vi "Dashboard Main.vi"() -> ()   [LabVIEW 2013]
uses:
  <vilib>/event_ctls.llb/eventvkey.ctl
  <vilib>/Rock Robotics/WPI/Dashboard/WPI_DashboardLogging Global.vi
  <vilib>/Utility/config.llb/Write Key (String).vi
  <vilib>/Utility/config.llb/Write Key (I32).vi
  <vilib>/Utility/config.llb/NI_LVConfig.lvlib
panel:
  out "Image Message":string="Timeout in Camera Communications"
  in  "Rec Mode":enum32{"Stop", "Record", "Playback"}(radio)
  in  "Dashboard Tab":T1(tab)
  out "Error":bool
  in  "Camera Settings":T2={"Frame Rate"=30, "Compression"=30, "Size"=1} {"Frame Rate" scale=1.0..30.0; "Size" items=["640x480", "320x240", "160x120"]}
  out "MotorSliders R":cluster{"MotorSlide1":dbl, "MotorSlide2":dbl} {"MotorSlide2" scale=-1.0..1.0 scale format="%#_2e"; "MotorSlide1" scale=-1.0..1.0 scale format="%#_2e"}
  out "MotorChart R":cluster{"Numeric":dbl, "Numeric":dbl}(graph)
  out "MotorSliders L":T3 {"MotorSlide4 2" scale=0.0..14.0 scale format="%#_2e"; "MotorSlide2" scale=-1.0..1.0 scale format="%#_2e"; "MotorSlide1" scale=-1.0..1.0 scale format="%#_2e"}
  out "MotorChart L":T4(graph)
  out "JS1 Z":dbl(slide) scale=-1.0..1.0 scale format="%#_2e"
  out "Joystick 1":cluster{"X":dbl, "Y":dbl}[](graph)
  out "JS Buttons 1":T5
  out "JS2 Z":dbl(slide) scale=-1.0..1.0 scale format="%#_2e"
  out "Joystick 2":cluster{"X":dbl, "Y":dbl}[](graph)
  out "JS Buttons 2":T5
  out "Mode":T6(ring)=enum."Auto Disabled"
  out "Camera IP":string
  in  "DB Camera Config":bool
  out "fps":dbl format="%#.1g"
  out "Mbps":dbl format="%#.1g"
  out "Mbps 2":bool
  in  "Test Slider":dbl(slide) scale=0.0..100.0 scale format="%#_3g"
  in  "On/Off":bool caption="Solenoid"
  in  "Test Name":u16(ring) items=["Select the test to run...", "Example Test", "-------------------------------", "List of tests is built in robot code.", "Replace with your own automated tests."]
  in  "Test Tree":string(tree)
  in  "Motor":cluster{"Value":dbl, "Enable":bool} {"Value" scale=-1.0..1.0 scale format="%#_3g"}
  out "Progress":T7 {"Test Progress" scale=0.0..100.0}
  in  "Rev/Fwd":cluster{"Forward":bool, "Reverse":bool}
  in  "Test Ring":u16(ring) items=["Auto", "Fixed indoor", "Fixed outdoor 1", "Fixed outdoor 2", "Fixed fluorescent 1", "Fixed fluorescent 2", "Hold current"]
  in  "Listbox":i32(listbox)
  out "Tree":string(tree)
  out "Errors":T8(array[cluster])
  out "Camera Image":T9(plugin-control)
  in  "Enable":bool
  # "Left"
  # "Front"
  # "Right"
  # "Battery"
  # "Customize by placing controls and indicators here and name to\nmatch Dashboard Variables on robot."
  # "This tab is a great place for autonomous settings and validation.\nCustomize by placing controls and indicators here and name to\nmatch Dashboard Variables on robot."
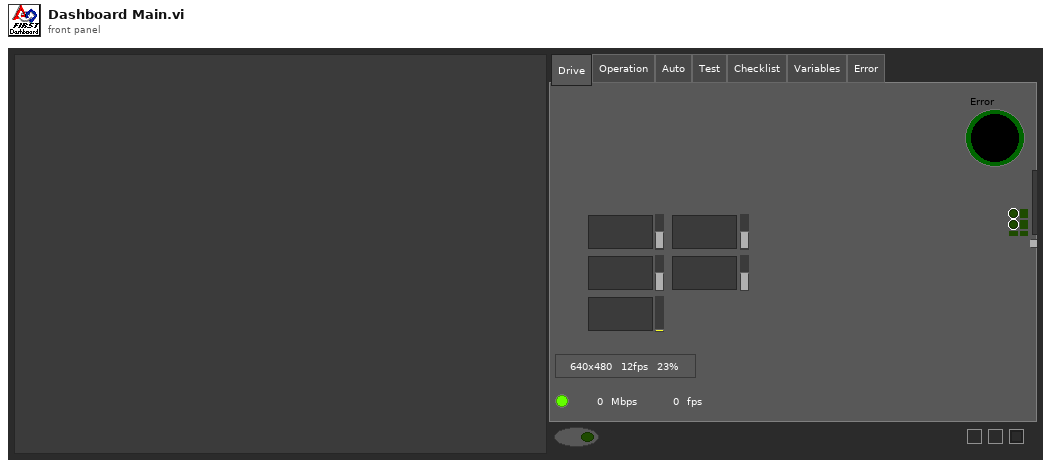
[diagram p1: front panel]
types:
  T1 = enum32{"Drive", "Operation", "Auto", "Test", "Checklist", "Variables", "Error"}
  T2 = cluster{"Frame Rate":i32, "Compression":i32, "Size":u16}
  T3 = cluster{"MotorSlide1":dbl, "MotorSlide2":dbl, "MotorSlide4 2":dbl}
  T4 = cluster{"Numeric":dbl, "Numeric":dbl, "Battery":sgl}
  T5 = cluster{bool, bool, bool, bool, bool, bool, bool, bool, bool, bool, bool, bool}
  T6 = enum8{"Tele-Op Disabled", "Tele-Op Enabled", "Auto Disabled", "Auto Enabled", "Test Disabled", "Test Enabled", ""}
  T7 = cluster{"Test Progress":u8, "Test Progress Text":string}
  T8 = cluster{"status":bool, "code":i32, "location":string, "source":string}[]
  T9 = typedef "IMAQ Image.ctl" = refnum<image>
  T10 = enum32{"Drive", "Operation", "Auto", "Test", "Checklist", "Variables"}
  T11 = typedef "Image Type" = u32
  T12 = cluster{"Digital Inputs":bool[], "Digital Outputs":bool[]}
  T13 = cluster{"Competition mode":bool, "Robot Link":bool, "Autonomous":bool, "Enabled":bool, "E-Stop":bool, "Simulated":bool, "TestMode":bool, "Docked Window":bool}
  T14 = cluster{"Boolean":bool, "Numeric":i32, "String":string, "String":string}[]
  T15 = cluster{"Boolean Array[0]":bool, "Boolean Array[1]":bool, "Boolean Array[2]":bool, "Boolean Array[3]":bool, "Boolean Array[4]":bool, "Boolean Array[5]":bool, "Boolean Array[6]":bool, "Boolean Array[7]":bool, "Boolean Array[8]":bool, "Boolean Array[9]":bool, "Boolean Array[10]":bool, "Boolean Array[11]":bool}
  T16 = typedef "NI_LVConfig.lvlib/Config Data RefNum.ctl" = refnum<k1>
  T17 = typedef "eventvkey.ctl" = enum16{"ASCII", "Enter", "Return", "Shift", "Ctrl", "Alt", "Cmd", "Opt", "Caps", "NumLock", "Clear", "Break", "Up", "Down", "Left", "Right", "Insert", "Delete", "Home", "End", "PageUp", "PageDown", "Escape", "Help", "Pause", "ScrollLock", "F1", "F2", "F3", "F4", "F5", "F6", "F7", "F8", "F9", "F10", "F11", "F12", "F13", "F14", "F15", "F16", "F17", "F18", "F19", "F20", "F21", "F22", "F23", "F24", "Play", "VolumeUp", "VolumeDown", "Mute", "Two Byte Char"}
  T18 = cluster{"Image Size":bool, "Image Type":bool, "Pixel Value":bool, "ROI Information":bool, "Zoom Factor":bool}
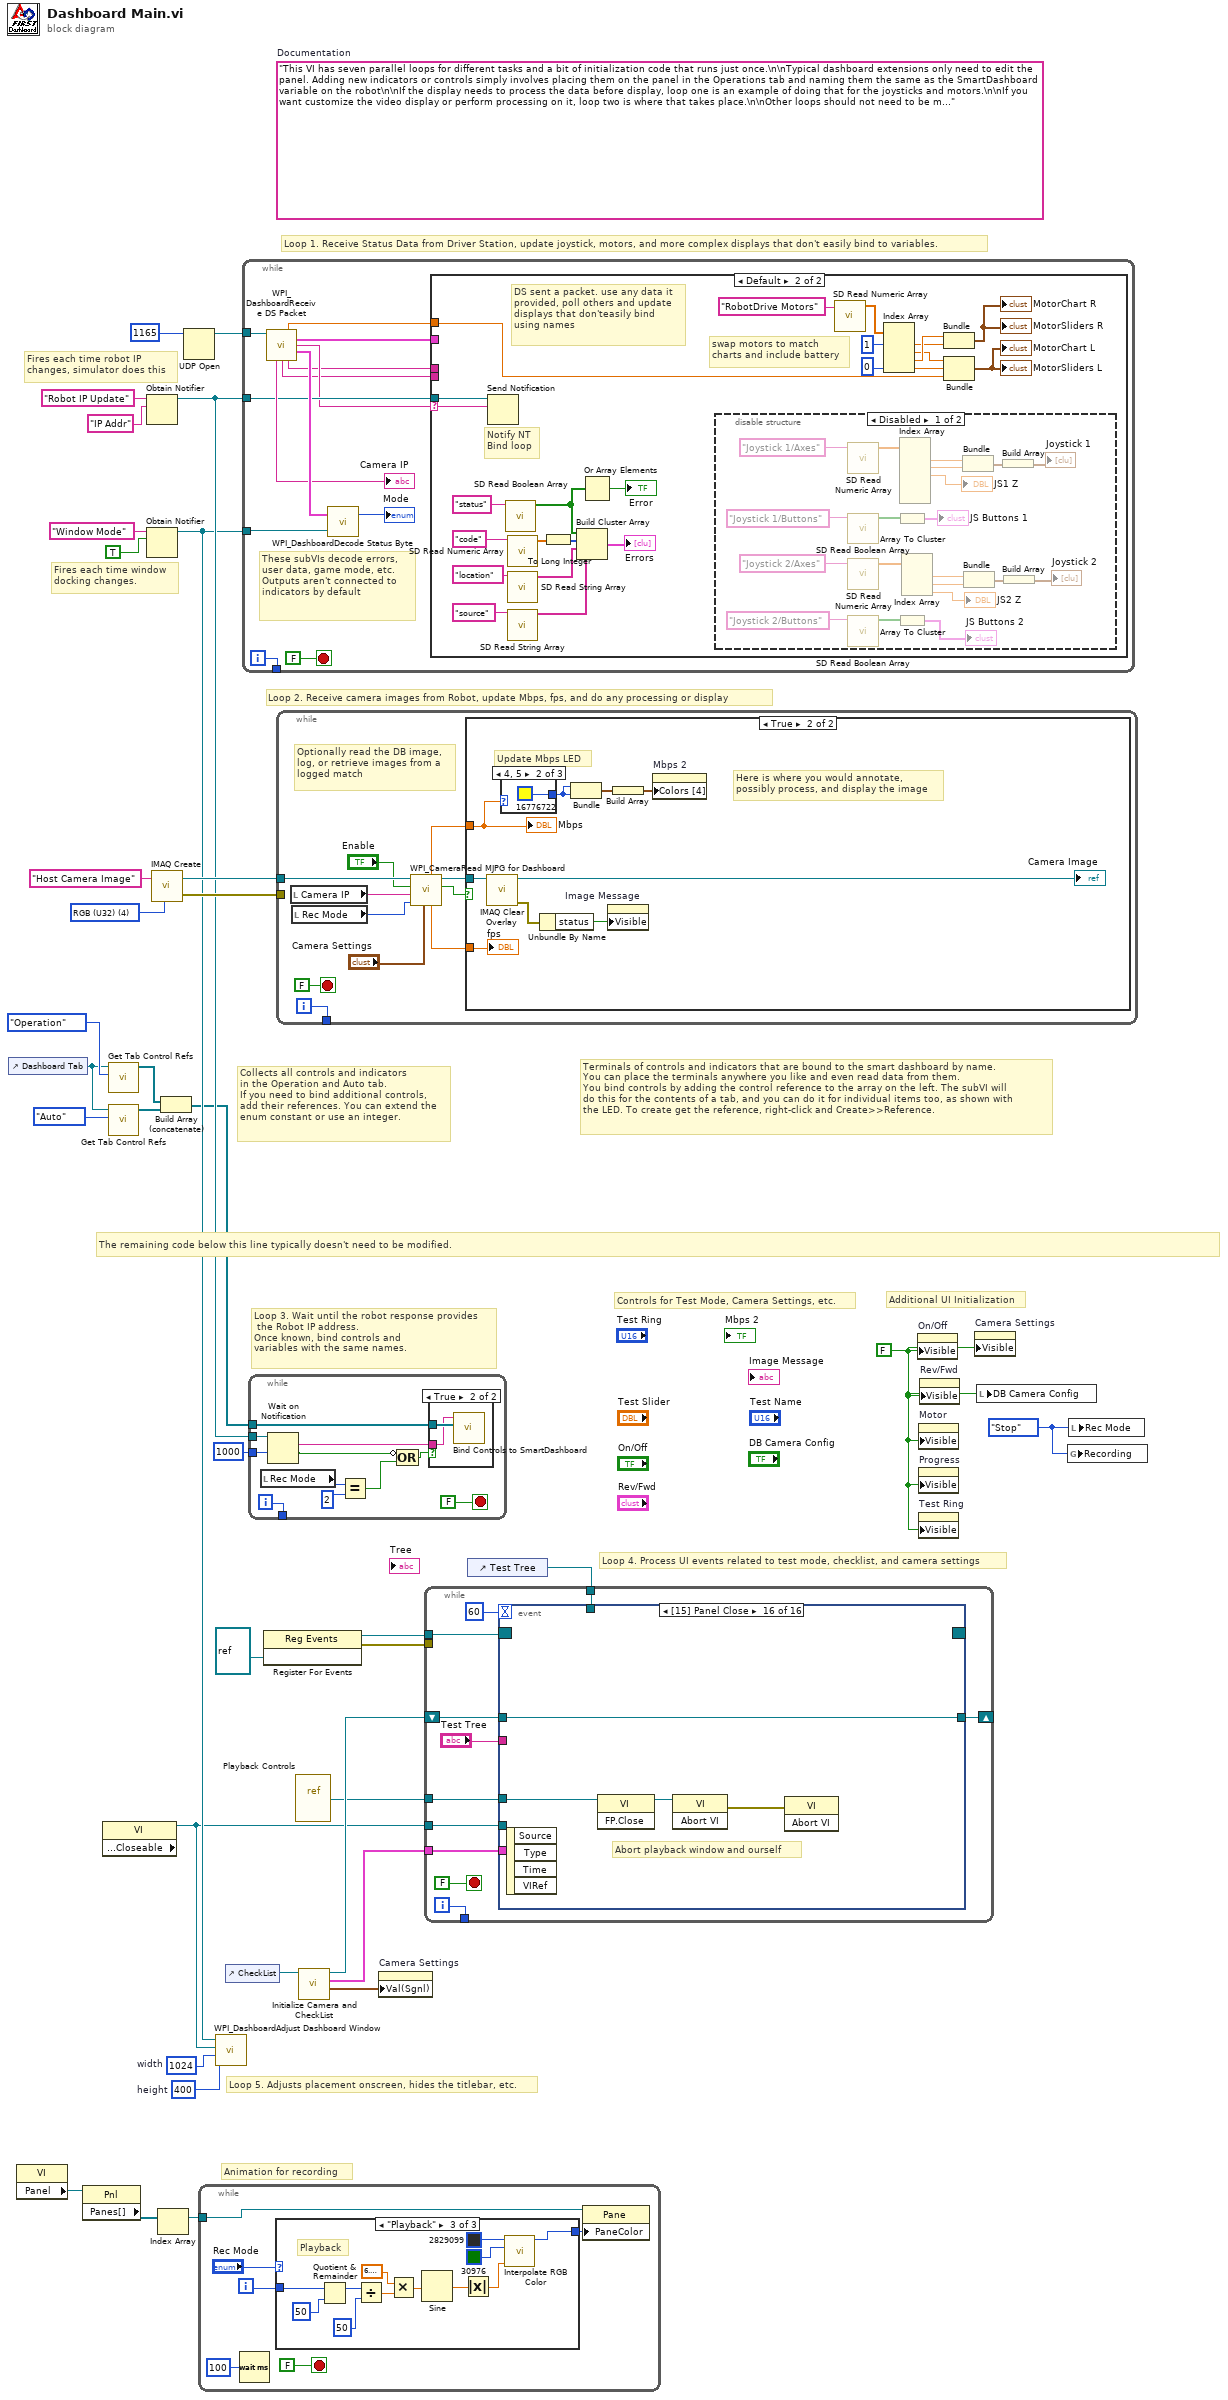
[diagram p0: block diagram]
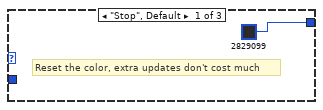
[diagram p2: hidden frame]
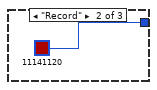
[diagram p3: hidden frame]
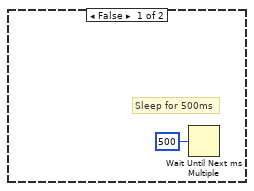
[diagram p5: hidden frame]
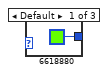
[diagram p6: hidden frame]
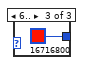
[diagram p7: hidden frame]
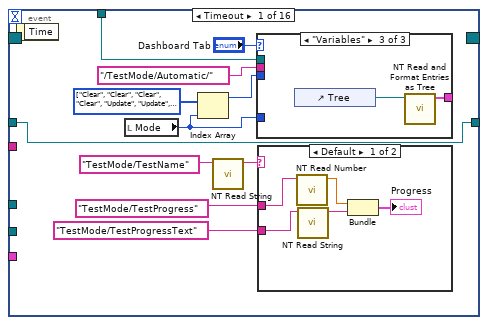
[diagram p8: hidden frame]
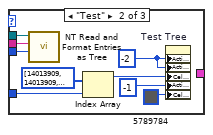
[diagram p10: hidden frame]
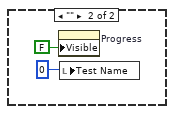
[diagram p11: hidden frame]
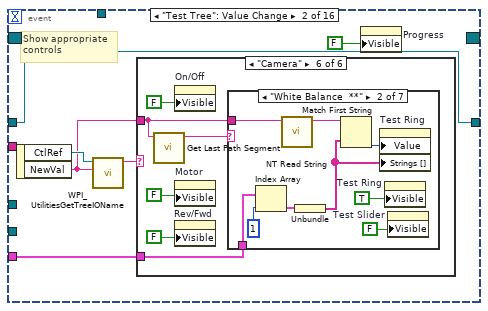
[diagram p12: hidden frame]
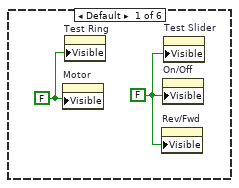
[diagram p13: hidden frame]
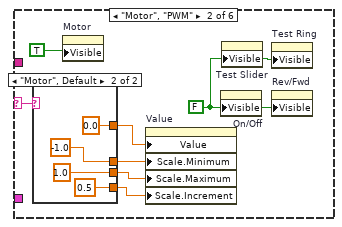
[diagram p14: hidden frame]
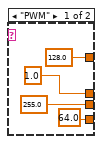
[diagram p15: hidden frame]
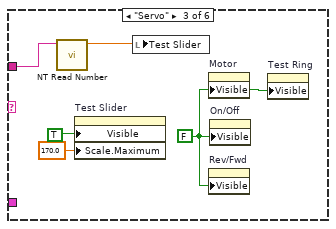
[diagram p16: hidden frame]
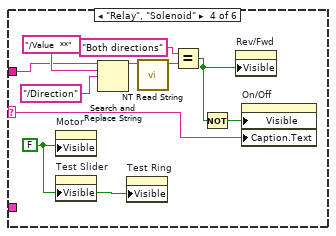
[diagram p17: hidden frame]
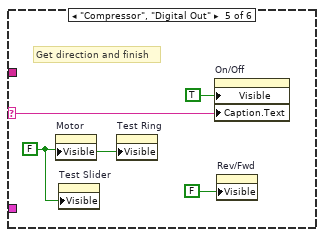
[diagram p18: hidden frame]
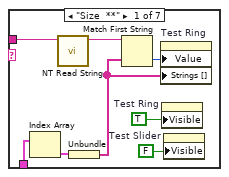
[diagram p19: hidden frame]
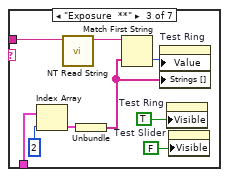
[diagram p20: hidden frame]
diagram:
  w7 = enum32{"Stop", "Record", "Playback"}."Stop" ("Rec Mode")
  w10 = 400  # height
  w11 = 1024  # width
  w24 = FALSE ("Visible")
  (unwired) "This VI has seven parallel loops for different tasks and a bit of initialization code that runs just once.\n\nTypical dashboard extensions only need to edit the panel. Adding new indicators or controls simply involves placing them on the panel in the Operations tab and naming them the same as the SmartDashboard variable on the robot\n\nIf the display needs to process the data before display, loop one is an example of doing that for the joysticks and motors.\n\nIf you want customize the video display or perform processing on it, loop two is where that takes place.\n\nOther loops should not need to be modified. They are pretty standard, and document the task they perform."  # Documentation
  w34 = T11 4 items=["Grayscale (U8)", "Grayscale (I16)", "Grayscale (SGL)", "Complex (CSG)", "RGB (U32)", "HSL (U32)", "RGB (U64)"] ("Image Type")
  # "Controls for Test Mode, Camera Settings, etc."
  # "Additional UI Initialization"
  # "Animation for recording"
  # "Fires each time robot IP\nchanges, simulator does this"
  # "Fires each time window\ndocking changes."
  # "Collects all controls and indicators\nin the Operation and Auto tab.\nIf you need to bind additional controls,\nadd their references. You can extend the\nenum constant or use an integer."
  # "The remaining code below this line typically doesn't need to be modified."
  # "Loop 4. Process UI events related to test mode, checklist, and camera settings"
  # "Terminals of controls and indicators that are bound to the smart dashboard by name.\nYou can place the terminals anywhere you like and even read data from them.\nYou bind controls by adding the control reference to the array on the left. The subVI will\ndo this for the contents of a tab, and you can do it for individual items too, as shown with\nthe LED. To create get the reference, right-click and Create>>Reference."
  # "Loop 3. Wait until the robot response provides\n the Robot IP address.\nOnce known, bind controls and\nvariables with the same names."
  # "Loop 5. Adjusts placement onscreen, hides the titlebar, etc."
  # "Loop 1. Receive Status Data from Driver Station, update joystick, motors, and more complex displays that don't easily bind to variables."
  # "Loop 2. Receive camera images from Robot, update Mbps, fps, and do any processing or display"
  n1 = control-ref of="Dashboard Tab"() -> (w5:refnum<vi>)
  n2 = property class="VI"() -> ("Panel"=w18:refnum<vi>)  [unwired: 2 in, 2 out]
  n3 = property class="Pnl"(reference=w18) -> ("Panes[]"=w19:refnum<vi>[])  [unwired: 1 in, 2 out]
  n4 = property class="VI" props=["Front Panel.Closeable"]() -> (reference out=w6:refnum<vi>)  [unwired: 2 in, 2 out]
  n5 = call <vilib>:"Get Tab Control Refs.vi"("Page Index"=T10."Operation" ("Dashboard Tab"), "TabControl in"=w5) -> ("ControlsOnPage"=w3:refnum<vi>[])  [unwired: 9 in]
  n6 = call <vilib>:"Get Tab Control Refs.vi"("Page Index"=T10."Auto" ("Dashboard Tab"), "TabControl in"=w5) -> ("ControlsOnPage"=w4:refnum<vi>[])  [unwired: 9 in]
  n7 = Obtain Notifier(name (unnamed)="Robot IP Update", notification data type="IP Addr" ("name (unnamed)")) -> (notifier out=w28:refnum<notifier>)  [unwired: 2 in, 2 out]
  n8 = Obtain Notifier(name (unnamed)="Window Mode", notification data type=TRUE) -> (notifier out=w9:refnum<notifier>)  [unwired: 2 in, 2 out]
  n9 = call "IMAQ Create"("Image Name"="Host Camera Image", "Image Type"=w34) -> ("New Image"=w32:T9, "error out"=w31:errorcluster)  [unwired: 2 in, 1 out]
  n10 = Index Array(array=w19) -> (element=w17:refnum<vi>)  [unwired: 1 in]
  n11 = Build Array (concatenate)(w3, w4) -> (w2:refnum<vi>[])
  n12 = UDP Open(11:u16 1165 ("port")) -> (port=w35:refnum<k16>)  [unwired: 2 in, 4 out]
  n13 = while {
    tunnel: w17 -> [w38]
    i -> [w41]
    stop <- FALSE stop-if-true
    n14 = Wait (ms)(milliseconds to wait=u32 100) -> ()  [unwired: 1 out]
    n15 = case shown="\"Playback\"" "Rec Mode" {
      tunnel: w41 -> [_ _ w56]
      tunnel: [u32 2829099 ("Base Color") u32 11141120 ("Target Color") w45] -> w37
      frame "Stop", Default {
        # "Reset the color, extra updates don't cost much"
      }
      frame "Record" {
      }
      frame "Playback" {
        # "Playback"
        n16 = Quotient & Remainder(x=w56, y=u32 50 ("milliseconds to wait")) -> (x-y*floor(x/y)=w52:u32)  [unwired: 1 out]
        n17 = Divide(x=w52, y=u32 50 ("milliseconds to wait")) -> (x/y=w49:dbl)
        n18 = Multiply(x=6.283185307179586, y=w49) -> (x*y=w54:dbl)
        n19 = Sine(x=w54) -> (sin(x)=w53:dbl)
        n20 = Absolute Value(x=w53) -> (abs(x)=w46:dbl)
        n21 = call "Interpolate RGB Color.vi"("Proportion"=w46, "Target Color"=u32 30976, "Base Color"=u32 2829099) -> ("Result Color"=w45:u32)  [unwired: 8 in]
      }
    }
    n22 = property class="Pane"(reference=w38, "PaneColor"=w37) -> ()  [unwired: 1 in, 2 out]
  }
  n23 = call <vilib>:"WPI_DashboardAdjust Dashboard Window.vi"("height"=w10, "width"=w11, "reference in"=w6, "Notifier in"=w9) -> ()  [unwired: 8 in]
  n24 = control-ref of="CheckList"() -> (w8:refnum<vi>)
  n25 = while {
    tunnel: w35 -> [w67]
    tunnel: w28 -> [w62]
    tunnel: w9 -> [w66]
    tunnel: [w63] -> _
    i -> [w63]
    stop <- FALSE stop-if-true
    # "These subVIs decode errors, user data, game mode, etc.\nOutputs aren't connected to indicators by default"
    n26 = call <vilib>:"WPI_DashboardReceive DS Packet.vi"("Recv Socket"=w67) -> ("Battery"=w57:sgl, "Driver Station"=w58:T12, "Robot IP Address"=w61:string, "Status"=w68:T13, "Camera IP Address"=→"Camera IP":string, "Low Priority User Data"=w60:string, "High Priority User Data"=w59:string)  [unwired: 1 in, 7 out]
    n27 = call <vilib>:"WPI_DashboardDecode Status Byte.vi"("Window Mode Notifier"=w66, "Status"=w68) -> ("Mode"=→"Mode":T6)  [unwired: 1 out]
    n28 = case shown="Default" w61 {
      selector: w61 -> [_ w91]
      tunnel: w62 -> [_ w92]
      tunnel: w60 -> [_ _]
      tunnel: w59 -> [_ _]
      tunnel: w58 -> [_ _]
      tunnel: w57 -> [_ w90]
      frame "0.0.0.0" {
        # "DS not sending packets, or no robot exists yet.\nDon't poll the variables"
      }
      frame Default {
        # "Notify NT\nBind loop"
        # "DS sent a packet. use any data it\nprovided, poll others and update\ndisplays that don'teasily bind\nusing names"
        # "swap motors to match\ncharts and include battery"
        n29 = Send Notification(notification=w91, notifier=w92) -> ()  [unwired: 1 in, 2 out]
        n30 = call <vilib>:"SD Read Boolean Array.vi"("Name"="status") -> ("Boolean Array"=w71:bool[])  [unwired: 8 in, 2 out]
        n31 = call <vilib>:"SD Read Numeric Array.vi"("Name"="code") -> ("Numeric Array"=w80:dbl[])  [unwired: 8 in, 2 out]
        n32 = call <vilib>:"SD Read String Array.vi"("Name"="location") -> ("String Array"=w78:string[])  [unwired: 9 in, 1 out]
        n33 = call <vilib>:"SD Read String Array.vi"("Name"="source") -> ("String Array"=w73:string[])  [unwired: 9 in, 1 out]
        n34 = To Long Integer(number=w80) -> (32bit integer=w79:i32[])
        n35 = Build Cluster Array(w71, w79, w78, w73) -> (→"Errors":T14)
        n36 = Or Array Elements(Boolean array=w71) -> (logical OR=→"Error":bool)
        n37 = disable-structure shown="Disabled" {
          frame Disabled {
            n38 = call <vilib>:"SD Read Numeric Array.vi"("Name"="Joystick 1/Axes") -> ("Numeric Array"=w109:dbl[])  [unwired: 8 in, 2 out]
            n39 = call <vilib>:"SD Read Boolean Array.vi"("Name"="Joystick 1/Buttons") -> ("Boolean Array"=w111:bool[])  [unwired: 8 in, 2 out]
            n40 = call <vilib>:"SD Read Numeric Array.vi"("Name"="Joystick 2/Axes") -> ("Numeric Array"=w103:dbl[])  [unwired: 8 in, 2 out]
            n41 = call <vilib>:"SD Read Boolean Array.vi"("Name"="Joystick 2/Buttons") -> ("Boolean Array"=w102:bool[])  [unwired: 8 in, 2 out]
            n42 = Array To Cluster(array=w111) -> (cluster=→"JS Buttons 1":T15)
            n43 = Array To Cluster(array=w102) -> (cluster=→"JS Buttons 2":T15)
            n44 = Index Array(array=w109) -> (element #1=w106:dbl, element #2=w107:dbl, element #3=→"JS1 Z":dbl)  [unwired: 6 in, 3 out]
            n45 = Index Array(array=w103) -> (element #1=w98:dbl, element #2=w97:dbl, element #3=→"JS2 Z":dbl)  [unwired: 3 in]
            n46 = Bundle("Numeric"=w106, "Numeric"=w107) -> (w105:cluster{"Numeric":dbl, "Numeric":dbl})  [unwired: 1 in]
            n47 = Bundle("Numeric"=w98, "Numeric"=w97) -> (w99:cluster{"Numeric":dbl, "Numeric":dbl})  [unwired: 1 in]
            n48 = Build Array(w105) -> (→"Joystick 1":cluster{"Numeric":dbl, "Numeric":dbl}[])
            n49 = Build Array(w99) -> (→"Joystick 2":cluster{"Numeric":dbl, "Numeric":dbl}[])
          }
          frame Enabled {
          }
        }
        n50 = call <vilib>:"SD Read Numeric Array.vi"("Name"="RobotDrive Motors") -> ("Numeric Array"=w89:dbl[])  [unwired: 8 in, 2 out]
        n51 = Index Array(array=w89, index #1=1, index #4=0) -> (element #1=w85:dbl, element #2=w84:dbl, element #3=w86:dbl, element #4=w81:dbl)  [unwired: 2 in]
        n52 = Bundle("Numeric"=w86, "Numeric"=w85) -> (→"MotorChart R" →"MotorSliders R":cluster{"Numeric":dbl, "Numeric":dbl})  [unwired: 1 in]
        n53 = Bundle("Numeric"=w84, "Numeric"=w81, "Battery"=w90) -> (→"MotorChart L" →"MotorSliders L":T4)  [unwired: 1 in]
      }
    }
  }
  n54 = while {
    tunnel: w2 -> [w124]
    tunnel: w28 -> [w122]
    tunnel: [w120] -> _
    tunnel: u32 1000 ("milliseconds to wait") -> [w119]
    i -> [w120]
    stop <- FALSE stop-if-true
    n55 = local read "Rec Mode"() -> (w115:enum32{"Stop", "Record", "Playback"})
    n56 = Wait on Notification(notifier=w122, timeout in ms (-1)=w119) -> (notification=w121:string, timed out?=w117:bool)  [unwired: 2 in, 2 out]
    n57 = Equal?(x=w115, y=u16 2 ("Rec Mode")) -> (x = y?=w116:bool)
    n58 = Compound Arithmetic op=OR(invert w117, w116) -> (w118:bool)
    n59 = case shown="True" w118 {
      tunnel: w124 -> [_ w126]
      tunnel: w121 -> [_ w125]
      frame False {
      }
      frame True {
        n60 = call <vilib>:"Bind Controls to SmartDashboard.vi"("Bound Control Refs"=w126, "Server IP Address"=w125) -> ()  [unwired: 10 in]
      }
    }
  }
  n61 = register-events(refnum<vi> refnum) -> (reference out=w15:refnum<event-registration>, error out=w14:errorcluster)  [unwired: 2 in]
  n62 = while {
    tunnel: w32 -> [w135]
    tunnel: w31 -> [_]
    tunnel: [w136] -> _
    i -> [w136]
    stop <- FALSE stop-if-true
    # "Optionally read the DB image,\nlog, or retrieve images from a\nlogged match"
    n63 = local read "Camera IP"() -> (w128:string)
    n64 = local read "Rec Mode"() -> (w127:enum32{"Stop", "Record", "Playback"})
    n65 = call <vilib>:"WPI_CameraRead MJPG for Dashboard.vi"("Camera Settings"="Camera Settings", "Rec Mode"=w127, "Camera IP"=w128, "Enable"="Enable", "Refnum in"=w135) -> ("Active"=w132:bool, "Refnum out"=w134:T9, "FPS"=w131:dbl, "Bandwidth (Mbps)"=w130:dbl)  [unwired: 3 in]
    n66 = case shown="True" w132 {
      tunnel: w134 -> [_ w142]
      tunnel: w130 -> [_ w141]
      tunnel: w131 -> [_ w139]
      frame False {
        # "Sleep for 500ms"
        n67 = Wait Until Next ms Multiple(millisecond multiple=u32 500) -> ()  [unwired: 1 out]
      }
      frame True {
        # "Here is where you would annotate,\npossibly process, and display the image"
        # "Update Mbps LED"
        n68 = call "IMAQ Clear Overlay"("Image"=w142) -> ("error out"=w146:errorcluster, "Image Out"=→"Camera Image":T9)  [unwired: 2 in, 7 out]
        n69 = case shown="4, 5" w141 {
          tunnel: [u32 6618880 ("Color Box") u32 16776722 ("Color Box") u32 16716800 ("Color Box")] -> w143
          frame Default {
          }
          frame 4, 5 {
          }
          frame 6.. {
          }
        }
        n70 = Unbundle By Name(w146) -> ("status"=w147:bool)
        n71 = Bundle("Color Box"=w143, "Color Box"=w143) -> (w145:cluster{"Color Box":u32, "Color Box":u32})  [unwired: 1 out]
        n72 = property on="Image Message" class="Str"("Visible"=w147) -> ()  [unwired: 2 in, 2 out]
        n73 = Build Array(w145) -> (w144:cluster{"Color Box":u32, "Color Box":u32}[])
        n74 = property on="Mbps 2" class="Bool (strict)"("Colors [4]"=w144) -> ()  [unwired: 2 in, 2 out]
        "Mbps" <- w141
        "fps" <- w139
      }
    }
  }
  n75 = vi-ref "Playback Controls.vi"() -> (w16:refnum<vi>)
  n76 = call "Initialize Camera and CheckList.vi"("ListBox in"=w8) -> ("Cluster"=w22:cluster{"value":i32, "value":i32, "index":i32}, "Array"=w23:cluster{string[]}[], "File Refnum"=w21:T16)  [unwired: 8 in]
  n77 = property on="Camera Settings" class="Clust (strict)"("Val(Sgnl)"=w22) -> ()  [unwired: 2 in, 2 out]
  n78 = control-ref of="Test Tree"() -> (w20:refnum<vi>)
  n79 = while {
    tunnel: w23 -> [w158]
    shift-right: [w157] -> _
    shift-left: w21 -> [w156]
    tunnel: [w155] -> _
    tunnel: w20 -> [w154]
    tunnel: w16 -> [w153]
    tunnel: w15 -> [w152]
    tunnel: w14 -> [_]
    tunnel: w6 -> [w151]
    i -> [w155]
    stop <- FALSE stop-if-true
    n80 = event shown="[15] Panel Close" {
      selector: w152 -> [_ _ _ _ _ _ _ _ _ _ _ _ _ _ _ _]
      dyn-events: [_ _ _ _ _ _ _ _ _ _ _ _ _ w396 _ _] -> _
      timeout: u32 60 ("milliseconds to wait") -> [_ _ _ _ _ _ _ _ _ _ _ _ _ _ _ _]
      tunnel: w154 -> [w168 _ _ _ _ _ _ _ _ _ _ _ _ _ _ _]
      tunnel: "Test Tree" -> [_ _ _ _ _ _ _ _ w365 w373 w375 w379 w387 _ _ _]
      tunnel: w158 -> [_ w192 _ _ _ _ w329 w359 _ _ _ _ _ _ _ _]
      tunnel: [w162 w191 w290 w295 w303 w315 w328 w352 w364 w371 w374 w378 w386 w398 w412 w413] -> w157
      tunnel: w156 -> [w162 w191 w290 w295 w303 w315 w327 w352 w364 w371 w374 w378 w386 w398 w412 w413]
      tunnel: w153 -> [_ _ _ _ _ _ _ _ _ _ _ _ _ w399 _ w416]
      tunnel: w151 -> [_ _ _ _ _ _ _ _ _ _ _ _ _ w394 _ _]
      event Timeout {
        w167 = enum16{"Update", "Clear"}[] [enum."Clear", enum."Clear", enum."Clear", enum."Clear", enum."Update", enum."Update", enum."Clear"] items=["Update", "Clear"]
        n81 = event-data() -> ()  [unwired: 1 in, 1 out]
        n82 = local read "Mode"() -> (w165:T6)
        n83 = Index Array(array=w167, index=w165) -> (element=w166:enum16{"Update", "Clear"})
        n84 = call <vilib>:"NT Read String.vi"("Name"="TestMode/TestName") -> ("String"=w171:string)  [unwired: 9 in, 1 out]
        n85 = case shown="\"Variables\"" "Dashboard Tab" {
          tunnel: w168 -> [_ w181 _]
          tunnel: "/TestMode/Automatic/" ("Name Pattern") -> [_ w180 _]
          tunnel: w166 -> [_ w179 _]
          tunnel: w165 -> [_ w177 _]
          tunnel: [_ _ w183] -> _
          frame "Operation", Default {
          }
          frame "Test" {
            w176 = -2 ("Active Item:Row Number")
            n86 = call <vilib>:"NT Read and Format Entries as Tree.vi"("Operation"=w179, "Name Pattern"=w180, "Tree Refnum"=w181) -> ()  [unwired: 7 in, 2 out]
            n87 = Index Array(array=u32[] [14013909, 14013909, 14013909, 14013909, 14013909, 16777215, 14013909], index=w177) -> (element=w175:u32)
            n88 = property on="Test Tree" class="Tree (strict)"("Active Item Row Number"=w176, "ActiveColNum"=w176, "CellBG"=w175, "Active Item Row Number"=-1 ("Active Item:Row Number"), "CellBG"=u32 5789784 ("Color Box")) -> ()  [unwired: 2 in, 2 out]
          }
          frame "Variables" {
            n89 = control-ref of="Tree"() -> (w182:refnum<vi>)
            n90 = call <vilib>:"NT Read and Format Entries as Tree.vi"("Tree Refnum"=w182) -> ("Formatted Strings"=w183:cluster{"Name":string, "Value":string}[])  [unwired: 9 in, 1 out]
          }
        }
        n91 = case shown="Default" w171 {
          tunnel: "TestMode/TestProgress" ("Name") -> [w185 _]
          tunnel: "TestMode/TestProgressText" ("Name") -> [w184 _]
          frame Default {
            n92 = call <vilib>:"NT Read Number.vi"("Name"=w185) -> ("Numeric"=w186:dbl)  [unwired: 9 in, 1 out]
            n93 = call <vilib>:"NT Read String.vi"("Name"=w184) -> ("String"=w187:string)  [unwired: 9 in, 1 out]
            n94 = Bundle("Numeric"=w186, "String"=w187) -> (→"Progress":cluster{"Numeric":dbl, "String":string})  [unwired: 1 in]
          }
          frame "" {
            n95 = property on="Progress" class="Clust (strict)"("Visible"=FALSE) -> ()  [unwired: 2 in, 2 out]
            n96 = local write "Test Name"(u16 0) -> ()
          }
        }
      }
      event "Test Tree": Value Change {
        # "Show appropriate\ncontrols"
        n97 = event-data() -> ("CtlRef"=w195:refnum<vi>, "NewVal"=w193:string)  [unwired: 1 in]
        n98 = call <vilib>:"WPI_UtilitiesGetTreeIOName.vi"("NewVal"=w193, "TreeControl in"=w195) -> ("I/O Name"=w196:string)  [unwired: 9 in]
        n99 = case shown="\"Camera\"" w196 {
          selector: w196 -> [_ w203 _ w221 w230 _]
          tunnel: w193 -> [_ _ w218 w220 _ w237]
          tunnel: w192 -> [_ _ _ _ _ w236]
          frame Default {
            w198 = FALSE ("Visible")
            w197 = FALSE ("Visible")
            n100 = property on="Motor" class="Clust (strict)"("Visible"=w197) -> ()  [unwired: 2 in, 2 out]
            n101 = property on="Test Ring" class="Ring (strict)"("Visible"=w197) -> ()  [unwired: 2 in, 2 out]
            n102 = property on="Rev/Fwd" class="Clust (strict)"("Visible"=w198) -> ()  [unwired: 2 in, 2 out]
            n103 = property on="On/Off" class="Bool (strict)"("Visible"=w198) -> ()  [unwired: 2 in, 2 out]
            n104 = property on="Test Slider" class="Slide (strict)"("Visible"=w198) -> ()  [unwired: 2 in, 2 out]
          }
          frame "Motor", "PWM" {
            w204 = FALSE ("Visible")
            n105 = case shown="\"Motor\", Default" w203 {
              tunnel: [1.0 ("Value") -1.0 ("Value")] -> w202
              tunnel: [255.0 ("Value") 1.0 ("Value")] -> w201
              tunnel: [128.0 ("Value") 0.0 ("Value")] -> w200
              tunnel: [64.0 ("Value") 0.5 ("Value")] -> w199
              frame "PWM" {
              }
              frame "Motor", Default {
              }
            }
            n106 = property on="Motor" class="Clust (strict)"("Visible"=TRUE) -> ()  [unwired: 2 in, 2 out]
            n107 = property on="Value" class="Slide (strict)"("Value"=w200, "Scale.Minimum"=w202, "Scale.Maximum"=w201, "Scale.Increment"=w199) -> ()  [unwired: 2 in, 2 out]
            n108 = property on="On/Off" class="Bool (strict)"("Visible"=w204) -> ()  [unwired: 2 in, 2 out]
            n109 = property on="Test Slider" class="Slide (strict)"("Visible"=w204) -> ()  [unwired: 2 in, 2 out]
            n110 = property on="Test Ring" class="Ring (strict)"("Visible"=w204) -> ()  [unwired: 2 in, 2 out]
            n111 = property on="Rev/Fwd" class="Clust (strict)"("Visible"=w204) -> ()  [unwired: 2 in, 2 out]
          }
          frame "Servo" {
            w216 = FALSE ("Visible")
            n112 = call <vilib>:"NT Read Number.vi"("Name"=w218) -> ("Numeric"=w217:dbl)  [unwired: 9 in, 1 out]
            n113 = property on="Test Slider" class="Slide (strict)"("Visible"=TRUE, "Scale.Maximum"=170.0 ("Scale.Range:Maximum")) -> ()  [unwired: 2 in, 2 out]
            n114 = local write "Test Slider"(w217) -> ()
            n115 = property on="Motor" class="Clust (strict)"("Visible"=w216) -> ()  [unwired: 2 in, 2 out]
            n116 = property on="Rev/Fwd" class="Clust (strict)"("Visible"=w216) -> ()  [unwired: 2 in, 2 out]
            n117 = property on="On/Off" class="Bool (strict)"("Visible"=w216) -> ()  [unwired: 2 in, 2 out]
            n118 = property on="Test Ring" class="Ring (strict)"("Visible"=w216) -> ()  [unwired: 2 in, 2 out]
          }
          frame "Relay", "Solenoid" {
            w219 = FALSE ("Visible")
            n119 = property on="Motor" class="Clust (strict)"("Visible"=w219) -> ()  [unwired: 2 in, 2 out]
            n120 = property on="Test Slider" class="Slide (strict)"("Visible"=w219) -> ()  [unwired: 2 in, 2 out]
            n121 = Search and Replace String(input string=w220, search string="/Value  **", replace string="/Direction") -> (result string=w226:string)  [unwired: 5 in, 3 out]
            n122 = property on="Test Ring" class="Ring (strict)"("Visible"=w219) -> ()  [unwired: 2 in, 2 out]
            n123 = call <vilib>:"NT Read String.vi"("Name"=w226) -> ("String"=w224:string)  [unwired: 9 in, 1 out]
            n124 = Equal?(x="Both directions", y=w224) -> (x = y?=w222:bool)
            n125 = Not(x=w222) -> (.not. x?=w223:bool)
            n126 = property on="Rev/Fwd" class="Clust (strict)"("Visible"=w222) -> ()  [unwired: 2 in, 2 out]
            n127 = property on="On/Off" class="Bool (strict)"("Visible"=w223, "Caption.Text"=w221) -> ()  [unwired: 2 in, 2 out]
          }
          frame "Compressor", "Digital Out" {
            w229 = FALSE ("Visible")
            # "Get direction and finish"
            n128 = property on="Motor" class="Clust (strict)"("Visible"=w229) -> ()  [unwired: 2 in, 2 out]
            n129 = property on="Test Slider" class="Slide (strict)"("Visible"=w229) -> ()  [unwired: 2 in, 2 out]
            n130 = property on="Test Ring" class="Ring (strict)"("Visible"=w229) -> ()  [unwired: 2 in, 2 out]
            n131 = property on="On/Off" class="Bool (strict)"("Visible"=TRUE, "Caption.Text"=w230) -> ()  [unwired: 2 in, 2 out]
            n132 = property on="Rev/Fwd" class="Clust (strict)"("Visible"=FALSE) -> ()  [unwired: 2 in, 2 out]
          }
          frame "Camera" {
            n133 = call <vilib>:"Get Last Path Segment.vi"("String in"=w237) -> ("String out"=w238:string)  [unwired: 10 in]
            n134 = property on="On/Off" class="Bool (strict)"("Visible"=FALSE) -> ()  [unwired: 2 in, 2 out]
            n135 = property on="Motor" class="Clust (strict)"("Visible"=FALSE) -> ()  [unwired: 2 in, 2 out]
            n136 = property on="Rev/Fwd" class="Clust (strict)"("Visible"=FALSE) -> ()  [unwired: 2 in, 2 out]
            n137 = case shown="\"White Balance  **\"" w238 {
              tunnel: w237 -> [w244 w253 w262 w271 w280 _ w286]
              tunnel: w236 -> [w242 w250 w259 w268 w277 _ _]
              frame "Size  **" {
                n138 = Index Array(array=w242) -> (element=w241:cluster{string[]})  [unwired: 1 in]
                n139 = call <vilib>:"NT Read String.vi"("Name"=w244) -> ("String"=w243:string)  [unwired: 9 in, 1 out]
                n140 = Unbundle(w241) -> (w239:string[])
                n141 = Match First String(2:w239, 3:w243) -> (0:w240:i32)  [unwired: 1 out]
                n142 = property on="Test Ring" class="Ring (strict)"("Value"=w240, "Strings []"=w239) -> ()  [unwired: 2 in, 2 out]
                n143 = property on="Test Ring" class="Ring (strict)"("Visible"=TRUE) -> ()  [unwired: 2 in, 2 out]
                n144 = property on="Test Slider" class="Slide (strict)"("Visible"=FALSE) -> ()  [unwired: 2 in, 2 out]
              }
              frame "White Balance  **" {
                n145 = Index Array(array=w250, index=1) -> (element=w251:cluster{string[]})
                n146 = call <vilib>:"NT Read String.vi"("Name"=w253) -> ("String"=w252:string)  [unwired: 9 in, 1 out]
                n147 = Unbundle(w251) -> (w248:string[])
                n148 = Match First String(2:w248, 3:w252) -> (0:w247:i32)  [unwired: 1 out]
                n149 = property on="Test Ring" class="Ring (strict)"("Value"=w247, "Strings []"=w248) -> ()  [unwired: 2 in, 2 out]
                n150 = property on="Test Ring" class="Ring (strict)"("Visible"=TRUE) -> ()  [unwired: 2 in, 2 out]
                n151 = property on="Test Slider" class="Slide (strict)"("Visible"=FALSE) -> ()  [unwired: 2 in, 2 out]
              }
              frame "Exposure  **" {
                n152 = Index Array(array=w259, index=2) -> (element=w260:cluster{string[]})
                n153 = call <vilib>:"NT Read String.vi"("Name"=w262) -> ("String"=w261:string)  [unwired: 9 in, 1 out]
                n154 = Unbundle(w260) -> (w256:string[])
                n155 = Match First String(2:w256, 3:w261) -> (0:w257:i32)  [unwired: 1 out]
                n156 = property on="Test Ring" class="Ring (strict)"("Value"=w257, "Strings []"=w256) -> ()  [unwired: 2 in, 2 out]
                n157 = property on="Test Ring" class="Ring (strict)"("Visible"=TRUE) -> ()  [unwired: 2 in, 2 out]
                n158 = property on="Test Slider" class="Slide (strict)"("Visible"=FALSE) -> ()  [unwired: 2 in, 2 out]
              }
              frame "Exposure Priority  **" {
                n159 = Index Array(array=w268, index=3) -> (element=w269:cluster{string[]})
                n160 = call <vilib>:"NT Read String.vi"("Name"=w271) -> ("String"=w270:string)  [unwired: 9 in, 1 out]
                n161 = Unbundle(w269) -> (w265:string[])
                n162 = Match First String(2:w265, 3:w270) -> (0:w266:i32)  [unwired: 1 out]
                n163 = property on="Test Ring" class="Ring (strict)"("Value"=w266, "Strings []"=w265) -> ()  [unwired: 2 in, 2 out]
                n164 = property on="Test Ring" class="Ring (strict)"("Visible"=TRUE) -> ()  [unwired: 2 in, 2 out]
                n165 = property on="Test Slider" class="Slide (strict)"("Visible"=FALSE) -> ()  [unwired: 2 in, 2 out]
              }
              frame "Color Enable  **" {
                n166 = Index Array(array=w277, index=4) -> (element=w278:cluster{string[]})
                n167 = call <vilib>:"NT Read String.vi"("Name"=w280) -> ("String"=w279:string)  [unwired: 9 in, 1 out]
                n168 = Unbundle(w278) -> (w274:string[])
                n169 = Match First String(2:w274, 3:w279) -> (0:w275:i32)  [unwired: 1 out]
                n170 = property on="Test Ring" class="Ring (strict)"("Value"=w275, "Strings []"=w274) -> ()  [unwired: 2 in, 2 out]
                n171 = property on="Test Ring" class="Ring (strict)"("Visible"=TRUE) -> ()  [unwired: 2 in, 2 out]
                n172 = property on="Test Slider" class="Slide (strict)"("Visible"=FALSE) -> ()  [unwired: 2 in, 2 out]
              }
              frame Default {
                n173 = property on="Test Ring" class="Ring (strict)"("Visible"=FALSE) -> ()  [unwired: 2 in, 2 out]
                n174 = property on="Test Slider" class="Slide (strict)"("Visible"=FALSE) -> ()  [unwired: 2 in, 2 out]
              }
              frame "Brightness  **", "Color Level  **", "Compression  **", "FPS  **", "Sharpness  **" {
                n175 = call <vilib>:"NT Read Number.vi"("Name"=w286) -> ("Numeric"=w285:dbl)  [unwired: 9 in, 1 out]
                n176 = local write "Test Slider"(w285) -> ()
                n177 = property on="Test Slider" class="Slide (strict)"("Visible"=TRUE, "Scale.Maximum"=100.0 ("Scale.Range:Maximum")) -> ()  [unwired: 2 in, 2 out]
                n178 = property on="Test Ring" class="Ring (strict)"("Visible"=FALSE) -> ()  [unwired: 2 in, 2 out]
              }
            }
          }
        }
        n179 = property on="Progress" class="Clust (strict)"("Visible"=FALSE) -> ()  [unwired: 2 in, 2 out]
      }
      event "Test Name": Mouse Enter {
        # "Populate the ring with the list of tests"
        n180 = event-data() -> ()  [unwired: 1 in, 1 out]
        n181 = call <vilib>:"NT Read String Array.vi"("Name"="TestMode/TestList") -> ("String Array"=w294:string[])  [unwired: 9 in, 1 out]
        n182 = Build Array (concatenate)("Select the test to run...", w294) -> (w293:string[])
        n183 = property on="Test Name" class="Ring (strict)"("Strings []"=w293) -> ()  [unwired: 2 in, 2 out]
      }
      event "Test Name": Value Change {
        w296 = FALSE ("Visible")
        # "Tell the robot the test name to run"
        n184 = event-data() -> ("NewVal"=w300:u16)  [unwired: 1 in]
        n185 = property on="Test Name" class="Ring (strict)"() -> ("Strings []"=w301:string[])  [unwired: 2 in, 2 out]
        n186 = local write "Progress"(T7 {"Test Progress"=0, "Test Progress Text"=""} ("Progress")) -> ()
        n187 = Index Array(array=w301, index=w300) -> (element=w299:string)
        n188 = call <vilib>:"NT Write String.vi"("String"=w299, "Name"="TestMode/TestName") -> ()  [unwired: 9 in, 1 out]
        n189 = property on="Progress" class="Clust (strict)"("Visible"=TRUE) -> ()  [unwired: 2 in, 2 out]
        n190 = property on="Motor" class="Clust (strict)"("Visible"=w296) -> ()  [unwired: 2 in, 2 out]
        n191 = property on="Test Slider" class="Slide (strict)"("Visible"=w296) -> ()  [unwired: 2 in, 2 out]
        n192 = property on="On/Off" class="Bool (strict)"("Visible"=w296) -> ()  [unwired: 2 in, 2 out]
        n193 = property on="Rev/Fwd" class="Clust (strict)"("Visible"=w296) -> ()  [unwired: 2 in, 2 out]
        n194 = property on="Test Ring" class="Ring (strict)"("Visible"=w296) -> ()  [unwired: 2 in, 2 out]
      }
      event "Listbox": Double Click {
        n195 = event-data() -> ("PlatMods.Shift"=w304:bool, "Row"=w306:i32)  [unwired: 1 in]
        n196 = case shown="True" w304 {
          tunnel: w306 -> [w310 _]
          tunnel: 1 -> [w309 _]
          frame False {
            n197 = property on="Listbox" class="LstBox (strict)"() -> ("Item Symbols"=w308:i32[])  [unwired: 2 in, 2 out]
            n198 = Replace Array Subset(array=w308, new element=w309, index=w310) -> (w307:i32[])
            n199 = property on="Listbox" class="LstBox (strict)"("Item Symbols"=w307) -> ()  [unwired: 2 in, 2 out]
          }
          frame True {
            w311 = 0 ("Top Row")
            n200 = property on="Listbox" class="LstBox (strict)"() -> ("Number of Rows"=w313:u32)  [unwired: 2 in, 2 out]
            n201 = Initialize Array(0, w313) -> (w312:i32[])
            n202 = property on="Listbox" class="LstBox (strict)"("Top Row"=w311, "Value"=w311, "Item Symbols"=w312) -> ()  [unwired: 2 in, 2 out]
          }
        }
      }
      event "Listbox": Key Down {
        n203 = event-data() -> ("VKey"=w317:T17)  [unwired: 1 in]
        n204 = case shown="\"Left\", \"Right\"" w317 {
          selector: w317 -> [w322 _]
          tunnel: eventvkey."Left" ("VKey") -> [w320 _]
          frame "Left", "Right" {
            n205 = Equal?(x=w320, y=w322) -> (x = y?=w321:bool)
            n206 = Select(t=0, s=w321, f=1) -> (s? t:f=w323:i32)
            n207 = property on="Listbox" class="LstBox (strict)"() -> ("Item Symbols"=w326:i32[])  [unwired: 2 in, 2 out]
            n208 = Replace Array Subset(array=w326, new element=w323, index="Listbox") -> (w325:i32[])
            n209 = property on="Listbox" class="LstBox (strict)"("Item Symbols"=w325) -> ()  [unwired: 2 in, 2 out]
          }
          frame Default {
          }
        }
      }
      event "DB Camera Config": Value Change {
        n210 = event-data() -> ("NewVal"=w330:bool)  [unwired: 1 in]
        n211 = case shown="False" w330 {
          tunnel: w329 -> [w339 _]
          tunnel: [w332 w350] -> w328
          tunnel: w327 -> [w331 w350]
          frame False {
            w346 = "Camera"
            w349 = FALSE ("Visible")
            n212 = local read "Camera Settings"() -> (w338:T2)
            n213 = Index Array(array=w339) -> (element=w342:cluster{string[]})  [unwired: 1 in]
            n214 = Unbundle(w338) -> ("Frame Rate"=w337:i32, "Compression"=w336:i32, "Size"=w340:u16)
            n215 = Unbundle(w342) -> (w341:string[])
            n216 = Index Array(array=w341, index=w340) -> (element=w335:string)
            n217 = call-poly <vilib>:"Write Key.vi"("section"=w346, "value"=w335, "key"="Size", "refnum"=w331) -> ("refnum out"=w348:T16)  [unwired: 2 in, 5 out]
            n218 = call-poly <vilib>:"Write Key.vi"("section"=w346, "value"=w337, "key"="FrameRate", "refnum"=w348) -> ("refnum out"=w347:T16)  [unwired: 1 in, 6 out]
            n219 = property on="Camera Settings" class="Clust (strict)"("Visible"=w349) -> ()  [unwired: 2 in, 2 out]
            n220 = local write "DB Camera Config"(w349) -> ()
            n221 = call-poly <vilib>:"Write Key.vi"("section"=w346, "value"=w336, "key"="Compression", "refnum"=w347) -> ("refnum out"=w333:T16)  [unwired: 1 in, 6 out]
            n222 = call <vilib>:"Close Config Data.vi"("refnum"=w333) -> ("file path"=w334:path)  [unwired: 2 in, 8 out]
            n223 = call <vilib>:"Open Config Data.vi"("configuration file path"=w334) -> ("refnum"=w332:T16)  [unwired: 8 in, 2 out]
          }
          frame True {
            n224 = property on="Camera Settings" class="Clust (strict)"("Visible"=TRUE) -> ()  [unwired: 2 in, 2 out]
          }
        }
      }
      event "Camera Settings": Value Change {
        n225 = event-data() -> ("NewVal"=w363:T2)  [unwired: 1 in]
        n226 = Index Array(array=w359) -> (element=w358:cluster{string[]})  [unwired: 1 in]
        n227 = Unbundle(w363) -> ("Frame Rate"=w354:i32, "Compression"=w353:i32, "Size"=w356:u16)
        n228 = Unbundle(w358) -> (w357:string[])
        n229 = Index Array(array=w357, index=w356) -> (element=w355:string)
        n230 = Format Into String(format string="%s   %dfps   %d%%", w355, w354, w353) -> (resulting string=w360:string)  [unwired: 2 in, 1 out]
        n231 = Build Array(w360) -> (w361:string[])
        n232 = property on="DB Camera Config" class="Bool (strict)"("Strings [4]"=w361) -> ()  [unwired: 2 in, 2 out]
      }
      event "Motor.Enable": Value Change {
        n233 = event-data() -> ("NewVal"=w369:bool)  [unwired: 1 in]
        n234 = Unbundle("Motor") -> ("Value"=w368:dbl)  [unwired: 1 out]
        n235 = Select(t=w368, s=w369, f=0.0) -> (s? t:f=w366:dbl)
        n236 = call <vilib>:"NT Write Number.vi"("Numeric"=w366, "Name"=w365) -> ()  [unwired: 9 in, 1 out]
      }
      event "Test Slider": Value Change {
        n237 = event-data() -> ("NewVal"=w372:dbl)  [unwired: 1 in]
        n238 = call <vilib>:"NT Write Number.vi"("Numeric"=w372, "Name"=w373) -> ()  [unwired: 9 in, 1 out]
      }
      event "On/Off": Value Change {
        n239 = event-data() -> ("NewVal"=w377:bool)  [unwired: 1 in]
        n240 = Boolean To (0,1)(Boolean=w377) -> (0, 1=w376:i16)
        n241 = call <vilib>:"NT Write Number.vi"("Numeric"=w376, "Name"=w375) -> ()  [unwired: 9 in, 1 out]
      }
      event "Rev/Fwd": Value Change {
        n242 = event-data() -> ("NewVal.Forward"=w385:bool, "NewVal.Reverse"=w384:bool)  [unwired: 1 in]
        n243 = Boolean To (0,1)(Boolean=w385) -> (0, 1=w381:i16)
        n244 = Boolean To (0,1)(Boolean=w384) -> (0, 1=w383:i16)
        n245 = Negate(x=w383) -> (-x=w382:i16)
        n246 = Add(x=w381, y=w382) -> (x+y=w380:i16)
        n247 = call <vilib>:"NT Write Number.vi"("Numeric"=w380, "Name"=w379) -> ()  [unwired: 9 in, 1 out]
      }
      event "Test Ring": Value Change {
        n248 = event-data() -> ("NewVal"=w389:u16)  [unwired: 1 in]
        n249 = property on="Test Ring" class="Ring (strict)"() -> ("Strings []"=w390:string[])  [unwired: 2 in, 2 out]
        n250 = Index Array(array=w390, index=w389) -> (element=w388:string)
        n251 = call <vilib>:"NT Write String.vi"("String"=w388, "Name"=w387) -> ()  [unwired: 9 in, 1 out]
      }
      event "Rec Mode": Value Change {
        # "Update globals for recording mode and path to read log from.\nClear when logging and let NetworkTables set path for vision to\nuse."
        n252 = event-data() -> ("NewVal"=w400:enum32{"Stop", "Record", "Playback"})  [unwired: 1 in]
        n253 = global write "WPI_DashboardLogging Global.vi" "Logging Filename"(path "") -> ()
        n254 = case shown="\"Stop\", \"Record\"" w400 {
          tunnel: w399 -> [_ w402 w410]
          tunnel: [_ _ w409] -> w396
          tunnel: [_ _ w408] -> _
          tunnel: w394 -> [_ _ w406]
          tunnel: cluster{i32, i32} {-250, 170} -> [_ _ w405]
          tunnel: [_ _ T18 {"Image Size"=TRUE, "Image Type"=TRUE, "Pixel Value"=TRUE, "ROI Information"=TRUE, "Zoom Factor"=FALSE} ("Image Information Shown:All Elements")] -> w392
          tunnel: [_ _ TRUE ("Zoom Factor")] -> w391
          frame Default {
          }
          frame "Stop", "Record" {
            # "Place Window too"
            n255 = invoke class="VI" method="FP.Close"(reference=w402) -> (reference out=w401:refnum<vi>)  [unwired: 2 in, 2 out]
            n256 = invoke class="VI" method="Abort VI"(reference=w401) -> ()  [unwired: 2 in, 3 out]
          }
          frame "Playback" {
            n257 = call "Open Playback Panel.vi"("Offset"=w405, "DB VI Ref"=w406, "Playback in"=w410) -> ("Playback out"=w407:refnum<vi>)  [unwired: 8 in]
            n258 = register-events(w407) -> (reference out=w409:refnum<event-registration>, error out=w408:errorcluster)  [unwired: 2 in]
          }
        }
        n259 = global write "WPI_DashboardLogging Global.vi" "Recording"(w400) -> ()
        n260 = property on="Camera Image" class="ImageControl"("Image Information Shown"=w392, "Image Information Visible"=w391) -> ()  [unwired: 2 in, 2 out]
        n261 = call <vilib>:"WPI_DashboardNT Log FieldName Cache.vi"("Operation"=enum16{"Lookup/Add", "Index", "Clear"}."Clear") -> ()  [unwired: 8 in, 3 out]
      }
      event Panel Close {
        w411 = enum32{"Stop", "Record", "Playback"}."Stop" ("Rec Mode")
        n262 = event-data() -> ()  [unwired: 1 in, 4 out]
        n263 = local write "Rec Mode"(w411) -> ()
        n264 = global write "WPI_DashboardLogging Global.vi" "Recording"(w411) -> ()
      }
      event Panel Close {
        # "Abort playback window and ourself"
        n265 = event-data() -> ()  [unwired: 1 in, 4 out]
        n266 = invoke class="VI" method="FP.Close"(reference=w416) -> (reference out=w415:refnum<vi>)  [unwired: 2 in, 2 out]
        n267 = invoke class="VI" method="Abort VI"(reference=w415) -> (error out=w414:errorcluster)  [unwired: 2 in, 2 out]
        n268 = invoke class="VI" method="Abort VI"(error in=w414) -> ()  [unwired: 2 in, 3 out]
      }
    }
  }
  n269 = property on="On/Off" class="Bool (strict)"("Visible"=w24) -> ()  [unwired: 2 in, 2 out]
  n270 = property on="Motor" class="Clust (strict)"("Visible"=w24) -> ()  [unwired: 2 in, 2 out]
  n271 = property on="Progress" class="Clust (strict)"("Visible"=w24) -> ()  [unwired: 2 in, 2 out]
  n272 = property on="Test Ring" class="Ring (strict)"("Visible"=w24) -> ()  [unwired: 2 in, 2 out]
  n273 = property on="Rev/Fwd" class="Clust (strict)"("Visible"=w24) -> ()  [unwired: 2 in, 2 out]
  n274 = property on="Camera Settings" class="Clust (strict)"("Visible"=w24) -> ()  [unwired: 2 in, 2 out]
  n275 = local write "DB Camera Config"(w24) -> ()
  n276 = global write "WPI_DashboardLogging Global.vi" "Recording"(w7) -> ()
  n277 = local write "Rec Mode"(w7) -> ()
